vi "Configure IF Bandwith.vi"(8 "error in (no error)":errorcluster, 10 "IF BW [Hz]":dbl, 11 "VNA-Keysight PNA in":refnum<class "VNA-Keysight PNA.lvclass">) -> (0 "error out":errorcluster, 2 "IF BW used [Hz]":dbl, 3 "VNA-Keysight PNA out":refnum<class "VNA-Keysight PNA.lvclass">)   [LabVIEW 2020, in "VNA-Keysight PNA.lvclass"]
doc: "Configures the Intermidiate Frequency Bandwidth. \nIt chooses the closest supported bandwidth.\nIt returns the used IF BW."
uses:
  VNA-Keysight PNA.lvclass
  C:/Sandbox/Git_Sandbox/WiSpry Test Framework source code (LV20)/WiSpry Test Framework/Instruments/Instrument.lvclass
  C:/Sandbox/Git_Sandbox/WiSpry Test Framework source code (LV20)/WiSpry Test Framework/Instruments/Vector Network Analyzer/Vector Network Analyzer.lvclass
  Instrument.lvclass/Instrument.ctl
  Vector Network Analyzer.lvclass/Vector Network Analyzer.ctl
  Instrument.lvclass
  Vector Network Analyzer.lvclass
  <instrlib>/Keysight PNA Series/Keysight PNA Series.lvlib
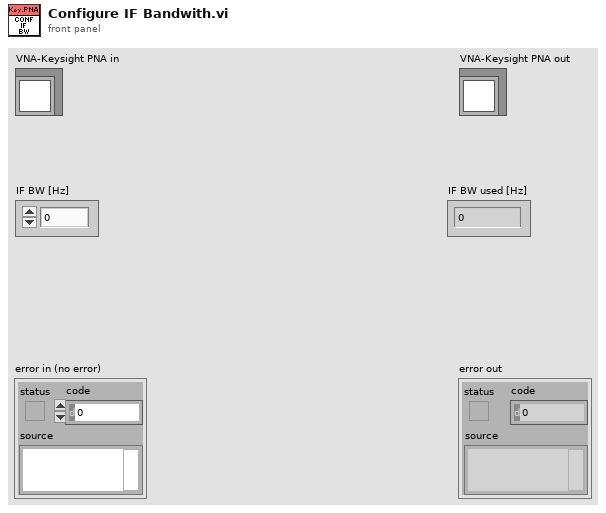
[diagram p1: front panel]
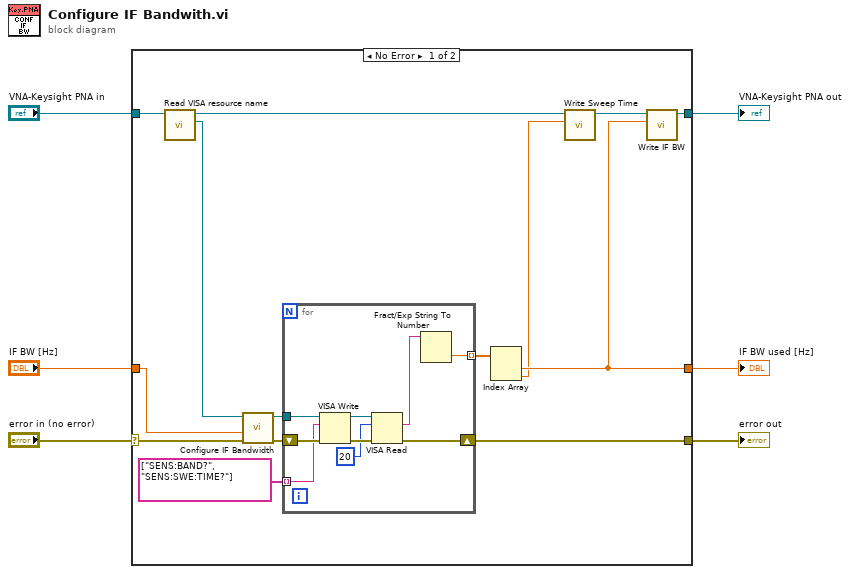
[diagram p0: block diagram]
diagram:
  n1 = case shown="No Error" "error in (no error)" {
    selector: "error in (no error)" -> [w18 w30]
    tunnel: [w19 w31] -> w4
    tunnel: "VNA-Keysight PNA in" -> [w20 w31]
    tunnel: [w13 w30] -> w5
    tunnel: [w8 w29] -> w2
    tunnel: "IF BW [Hz]" -> [w16 w29]
    frame No Error {
      n2 = call "Read VISA resource name.vi"("Instrument in"=w20) -> ("VISA resource name"=w17:refnum<visa-resource-name>, "Instrument out"=w12:refnum<class "VNA-Keysight PNA.lvclass">)  [unwired: 9 in]
      n3 = call <instrlib>:"Configure IF Bandwidth.vi"("error in (no error)"=w18, "Bandwidth (100000 Hz)"=w16, "VISA resource name"=w17) -> ("error out"=w14:errorcluster, "VISA resource name out"=w15:refnum<visa-resource-name>)  [unwired: 7 in]
      n4 = for {
        tunnel: w15 -> [w28]
        tunnel: [w22] -> w9 mode=indexing
        shift-right: [w25] -> w13
        shift-left: w14 -> [w26]
        tunnel: string[] ["SENS:BAND?", "SENS:SWE:TIME?"] -> [w21] mode=indexing
        n5 = VISA Write(VISA resource name=w28, write buffer=w21, error in (no error)=w26) -> (VISA resource name out=w27:refnum<visa-resource-name>)  [unwired: 2 out]
        n6 = VISA Read(VISA resource name=w27, byte count=u32 20, error in (no error)=w26) -> (read buffer=w23:string, error out=w25:errorcluster)  [unwired: 2 out]
        n7 = Fract/Exp String To Number(string=w23) -> (number=w22:dbl)  [unwired: 3 in, 1 out]
      }
      n8 = Index Array(array=w9) -> (element #1=w8:dbl, element #2=w7:dbl)  [unwired: 2 in]
      n9 = call "Write Sweep Time.vi"("Sweep Time"=w7, "Vector Network Analyzer in"=w12) -> ("Vector Network Analyzer out"=w11:refnum<class "VNA-Keysight PNA.lvclass">)  [unwired: 9 in]
      n10 = call "Write IF BW.vi"("IF BW"=w8, "Vector Network Analyzer in"=w11) -> ("Vector Network Analyzer out"=w19:refnum<class "VNA-Keysight PNA.lvclass">)  [unwired: 9 in]
    }
    frame Error {
    }
  }
  "error out" <- w5
  "VNA-Keysight PNA out" <- w4
  "IF BW used [Hz]" <- w2
